vi "flag_array.vi"() -> ()   [LabVIEW 2016]
panel:
  out "flags":bool[](array[boolean])
  # "Trigger State"
  # "Read Signal Param Change (output waveforms)"
  # "Reset  (stop inner loops)"
  # "Kill (stop outer loop and program)"
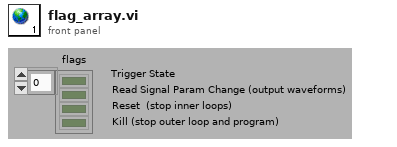
[diagram p1: front panel]
diagram:
